vi "Write Read Assert Factory.vi"(8 "error in (no error)":errorcluster, 11 "Assert Factory":refnum<class "Assert Factory.lvclass">) -> (0 "error out":errorcluster, 3 "Assert Factory":refnum<class "Assert Factory.lvclass">)   [LabVIEW 2009, in "Caraya.lvlib" / "Assert Factory Global.lvclass"]
uses:
  Assert Factory Global.lvclass
  Assert Factory/Assert Factory.lvclass
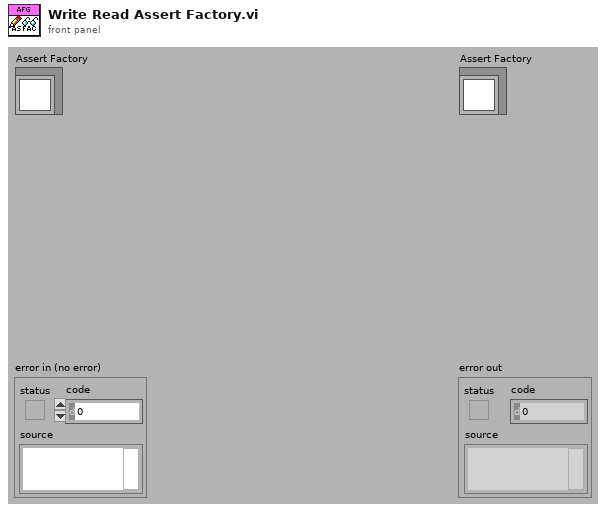
[diagram p1: front panel]
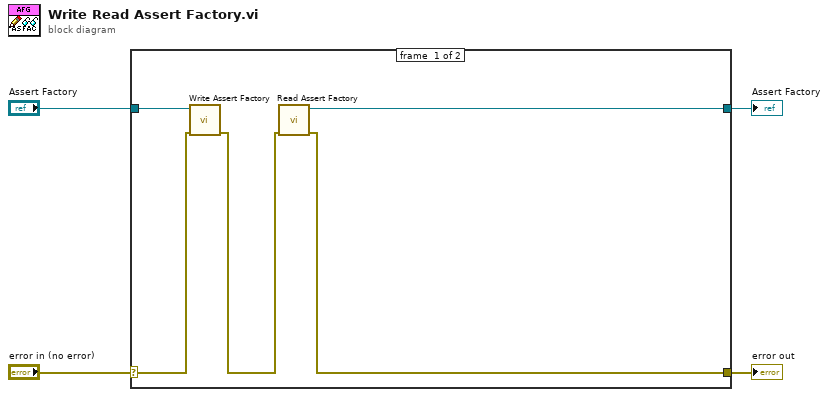
[diagram p0: block diagram]
diagram:
  n1 = case shown="No Error" "error in (no error)" {
    selector: "error in (no error)" -> [w8 w11]
    tunnel: [w6 w11] -> w3
    tunnel: [w5 w10] -> w1
    tunnel: "Assert Factory" -> [w9 w10]
    frame #0 {
      n2 = call "Write Assert Factory.vi"("error in (no error)"=w8, "Assert Factory"=w9) -> ("error out"=w7:errorcluster)  [unwired: 9 in]
      n3 = call "Read Assert Factory.vi"("error in (no error)"=w7) -> ("error out"=w6:errorcluster, "Assert Factory"=w5:refnum<class "Assert Factory.lvclass">)  [unwired: 9 in]
    }
    frame #1 {
    }
  }
  "error out" <- w3
  "Assert Factory" <- w1
